vi "Insert Plugin VI.vi"(7 "VI Name":T1, 8 "error in (no error)":errorcluster) -> (0 "error out":errorcluster)   [LabVIEW 2021, in "User Interface.lvlib"]
uses:
  User Interface.lvlib
  VI Name.ctl
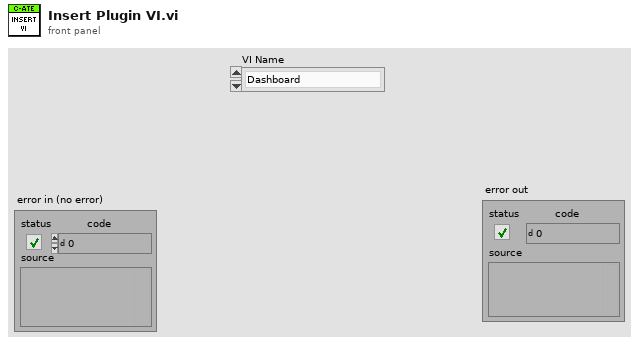
[diagram p1: front panel]
types:
  T1 = typedef "User Interface.lvlib/VI Name.ctl" = enum16{"Dashboard", "Maintenance", "Recipe", "Inst Configuration", "Testing", "Report"}
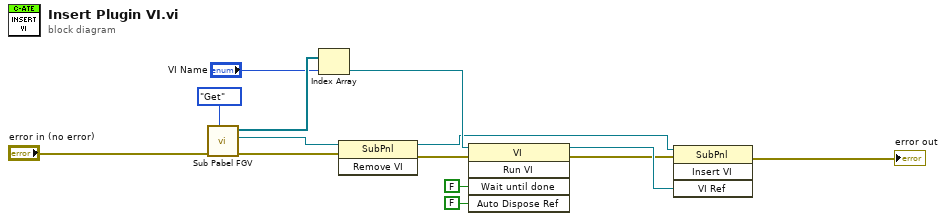
[diagram p0: block diagram]
diagram:
  n1 = call "Sub Pabel FGV.vi"("Command"=enum16{"Set", "Get"}."Get", "error in (no error)"="error in (no error)") -> ("error out"=w10:errorcluster, "Sub Panel"=w9:refnum<vi>, "Plug in VI"=w12:refnum<vi>[])  [unwired: 7 in]
  n2 = Index Array(array=w12, index="VI Name") -> (element=w7:refnum<vi>)
  n3 = invoke class="SubPnl" method="Remove VI"(reference=w9, error in=w10) -> (reference out=w2:refnum<vi>, error out=w8:errorcluster)  [unwired: 1 in, 1 out]
  n4 = invoke class="VI" method="Run VI"(reference=w7, error in=w8, "Wait until done"=FALSE ("Wait Until Done"), "Auto Dispose Ref"=FALSE ("Auto Dispose Reference")) -> (reference out=w4:refnum<vi>, error out=w3:errorcluster)  [unwired: 1 in, 3 out]
  n5 = invoke class="SubPnl" method="Insert VI"(reference=w2, error in=w3, "VI Ref"=w4) -> (error out=→"error out":errorcluster)  [unwired: 1 in, 3 out]
